vi "PDash - Duplicate DQMH Event.vi"(6 "Round Trip Broadcast Name":string, 7 "Destination Module":T1, 9 "New Event Name":string, 10 "Event Info (Existing)":T3={"Event VI Path"=path "", "Argument Path"=path "", "Wait Argument Path"=path "", "Event Arg Owner"=-1, "Event Name"="", "Type"=enum."Request"}, 11 "Source Module":T1) -> (0 "error out":errorcluster)   [LabVIEW 2019]
doc: "_____\nCreated using DQMH Event Scripter 7.1.0.1447."
uses:
  <vilib>/Delacor/Delacor QMH/Libraries/_Scripting Support/Module Info--cluster.ctl
  <vilib>/Delacor/Delacor QMH/Libraries/_Scripting Support/Module Type--enum.ctl
  <vilib>/Delacor/Delacor QMH/Libraries/_Scripting Support/Event Info (Existing)--cluster.ctl
  Program Files (x86)/National Instruments/LabVIEW 2019/project/Delacor/DQMH/_DQMH Remove Event/Event Type (All Permutations)--enum.ctl
  PantherDashboard Scripting Hooks/Panther Dasboard Scripting Hooks.lvlib
  <vilib>/Delacor/Delacor QMH/Libraries/_Scripting Support/dqmh_lib_DQMH Scripting Support.lvlib
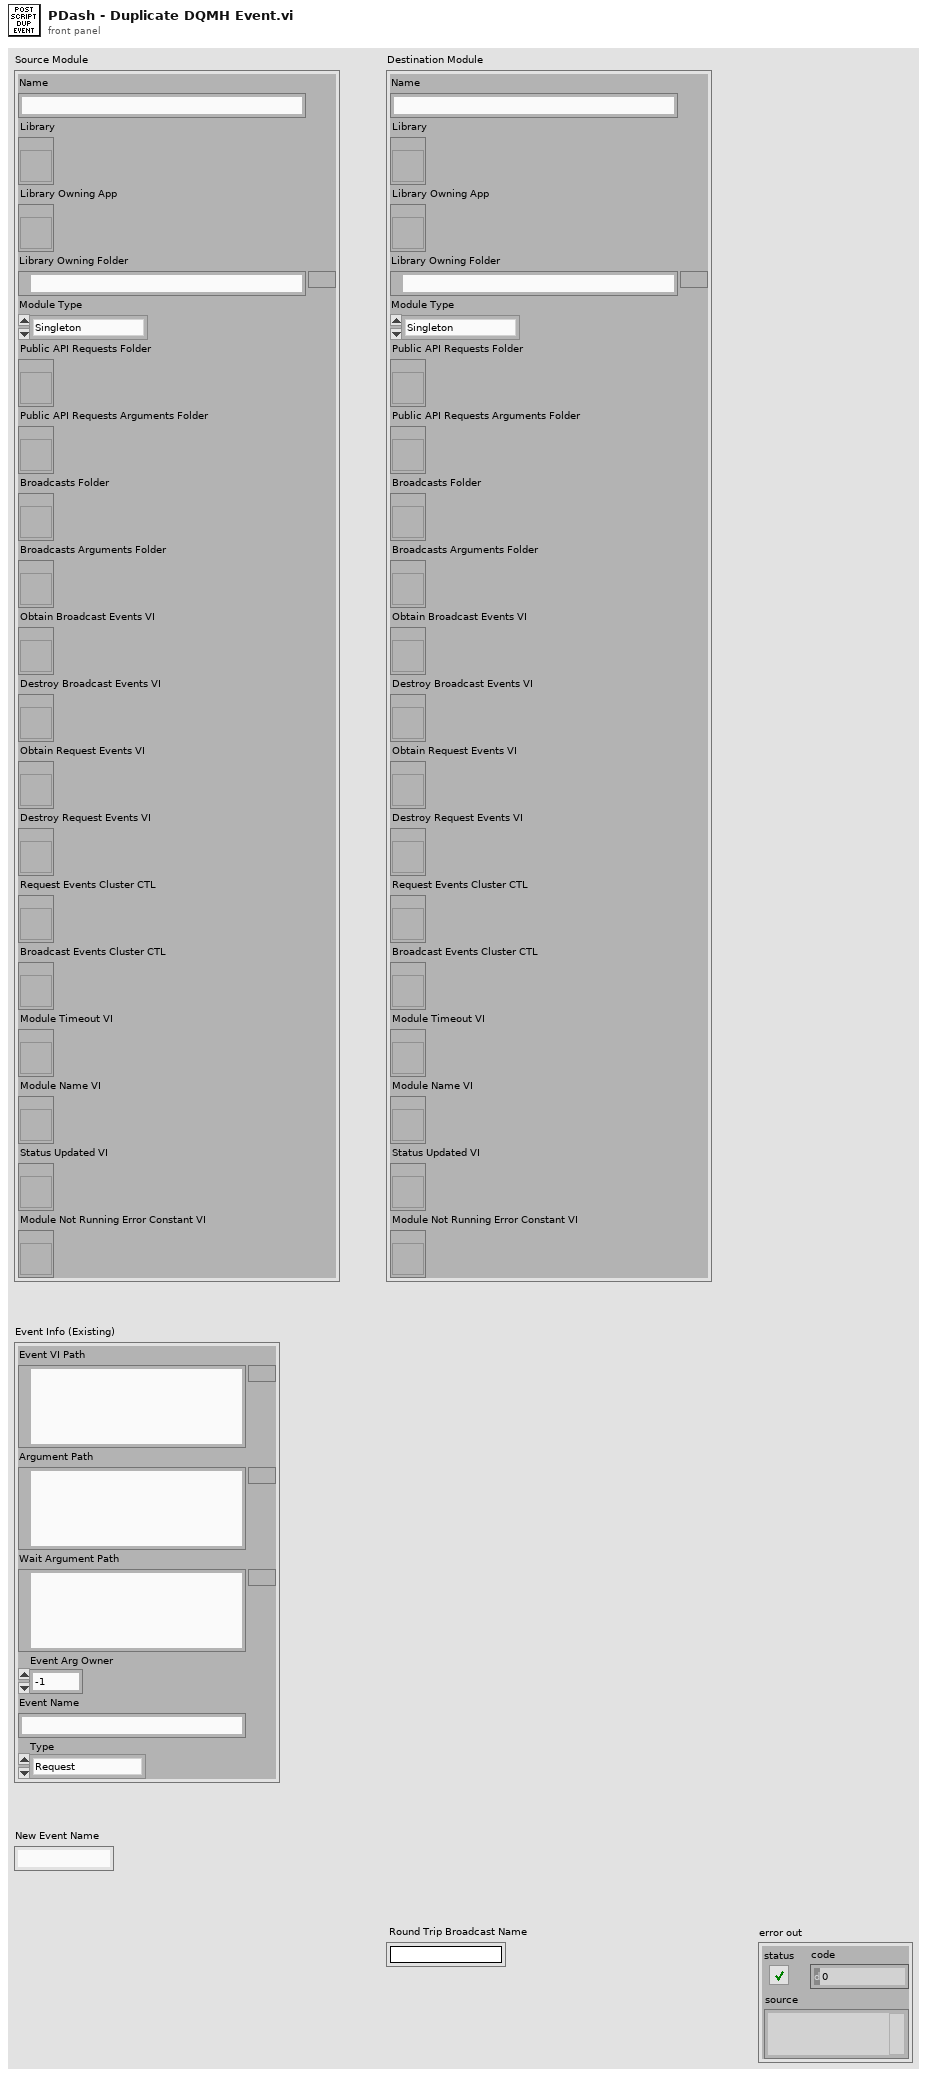
[diagram p1: front panel]
types:
  T1 = typedef "dqmh_lib_DQMH Scripting Support.lvlib/Module Info--cluster.ctl" = cluster{"Name":string, "Library":refnum<vi>, "Library Owning App":refnum<vi>, "Library Owning Folder":path, "Module Type":T2, "Public API Requests Folder":refnum<vi>, "Public API Requests Arguments Folder":refnum<vi>, "Broadcasts Folder":refnum<vi>, "Broadcasts Arguments Folder":refnum<vi>, "Obtain Broadcast Events VI":refnum<vi>, "Destroy Broadcast Events VI":refnum<vi>, "Obtain Request Events VI":refnum<vi>, "Destroy Request Events VI":refnum<vi>, "Request Events Cluster CTL":refnum<vi>, "Broadcast Events Cluster CTL":refnum<vi>, "Module Timeout VI":refnum<vi>, "Module Name VI":refnum<vi>, "Status Updated VI":refnum<vi>, "Module Not Running Error Constant VI":refnum<vi>}
  T2 = typedef "dqmh_lib_DQMH Scripting Support.lvlib/Module Type--enum.ctl" = enum16{"Singleton", "Cloneable"}
  T3 = typedef "dqmh_lib_DQMH Scripting Support.lvlib/Event Info (Existing)--cluster.ctl" = cluster{"Event VI Path":path, "Argument Path":path, "Wait Argument Path":path, "Event Arg Owner":i32, "Event Name":string, "Type":T4}
  T4 = typedef "dqmh_lib_DQMH Scripting Support.lvlib/Event Type (All Permutations)--enum.ctl" = enum16{"Request", "Broadcast", "Both", "Request (no Wait)", "Request and Wait", "Request (Private)", "Request (Local Instance)"}
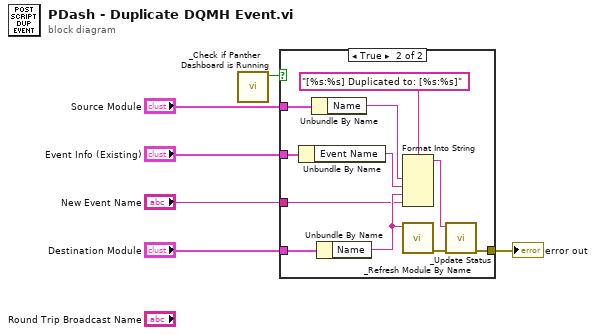
[diagram p0: block diagram]
diagram:
  n1 = call "_Check if Panther Dashboard is Running.vi"() -> ("Panther Dashboard is Running?"=w5:bool)  [unwired: 10 in, 1 out]
  n2 = case shown="True" w5 {
    tunnel: [_ w16] -> w6
    tunnel: "Destination Module" -> [_ w15]
    tunnel: "New Event Name" -> [_ w8]
    tunnel: "Source Module" -> [_ w13]
    tunnel: "Event Info (Existing)" -> [_ w12]
    frame False {
    }
    frame True {
      n3 = Unbundle By Name(w12) -> ("Event Name"=w10:string)
      n4 = Unbundle By Name(w13) -> ("Name"=w11:string)
      n5 = Unbundle By Name(w15) -> ("Name"=w9:string)
      n6 = Format Into String(format string="[%s:%s] Duplicated to: [%s:%s]", w11, w10, w9, w8) -> (resulting string=w14:string)  [unwired: 2 in, 1 out]
      n7 = call "_Refresh Module By Name.vi"("Module Name"=w9) -> ("error out"=w17:errorcluster)  [unwired: 10 in]
      n8 = call "_Update Status.vi"("error in"=w17, "Status"=w14) -> ("error out"=w16:errorcluster)  [unwired: 9 in]
    }
  }
  "error out" <- w6
